vi "NiXnet GetSubProperty.vi"(6 "contextId":T1, 8 "error in":errorcluster, 9 "timeout (ms)":i32=-1, 10 "Request Data":T3, 11 "gRPC ID":T1) -> (0 "error out":errorcluster, 2 "Response Data":T2, 3 "gRPC ID out":T1)   [LabVIEW 2025, in "xnet-grpc_client.lvlib"]
uses:
  xnet-grpc_client.lvlib
  <vilib>/gRPC/LabVIEW gRPC Library/Shared/grpcId.ctl
  RPC Messages/nixnet_grpc_GetSubPropertyRequest.ctl
  RPC Messages/nixnet_grpc_GetSubPropertyRequest_subproperty_id_enum/nixnet_grpc_GetSubPropertyRequest_subproperty_id_enum.lvclass
  RPC Messages/nidevice_grpc_Session.ctl
  RPC Messages/nixnet_grpc_GetSubPropertyResponse.ctl
  RPC Messages/nixnet_grpc_GetSubPropertyResponse_property_value/nixnet_grpc_GetSubPropertyResponse_property_value.lvclass
  RPC Messages/nixnet_grpc_GetSubPropertyResponse_Flat.ctl
  RPC Messages/nixnet_grpc_GetSubPropertyRequest_subproperty_id_enum/nixnet_grpc_GetSubPropertyRequest_subproperty_id_enum.lvclass/nixnet_grpc_GetSubPropertyRequest_subproperty_id_enum.ctl
  RPC Messages/nixnet_grpc_GetSubPropertyResponse_property_value/nixnet_grpc_GetSubPropertyResponse_property_value.lvclass/nixnet_grpc_GetSubPropertyResponse_property_value.ctl
  14035477-4c25-4107-8ed5-d0c4ef420ce5.vi
  RPC Messages/RichToFlatnidevice_grpc_Session.vi
  RPC Messages/nixnet_grpc_GetSubPropertyRequest_subproperty_id_enum/GetActiveFieldIndex.vi
  RPC Messages/nixnet_grpc_GetSubPropertyRequest_subproperty_id_enum/Getproperty_id.vi
  RPC Messages/nixnet_grpc_GetSubPropertyRequest_subproperty_id_enum/Getproperty_id_raw.vi
  <vilib>/gRPC/LabVIEW gRPC Library/Shared/TranslateGrpcError.vi
  <vilib>/gRPC/LabVIEW gRPC Library/Shared/Wait On Occurrence Wrapper.vi
  RPC Messages/nixnet_grpc_GetSubPropertyResponse_property_value/Setu32_scalar.vi
  RPC Messages/nixnet_grpc_GetSubPropertyResponse_property_value/Setstr.vi
  RPC Messages/nixnet_grpc_GetSubPropertyResponse_property_value/Setf64_scalar.vi
  <vilib>/gRPC/LabVIEW gRPC Library/Shared/Wait On Occurence.vi
  <vilib>/gRPC/LabVIEW gRPC Library/Server API/Server/Get Server DLL Path.vi
  <vilib>/Utility/error.llb/Error Cluster From Error Code.vi
  <vilib>/Utility/config.llb/Open Config Data.vi
  <vilib>/Utility/config.llb/Write Key.vi
  <vilib>/Utility/config.llb/Write Key (Boolean).vi
  <vilib>/Utility/config.llb/Not A Config Data Refnum.vi
  <vilib>/Utility/config.llb/Read Key.vi
  <vilib>/Utility/config.llb/Read Key (Boolean).vi
  <vilib>/Utility/config.llb/Close Config Data.vi
  RPC Messages/nixnet_grpc_GetSubPropertyResponse_property_value/GetActiveFieldName.vi
  <vilib>/gRPC/LabVIEW gRPC Library/grpc-lvsupport-release.lvlib
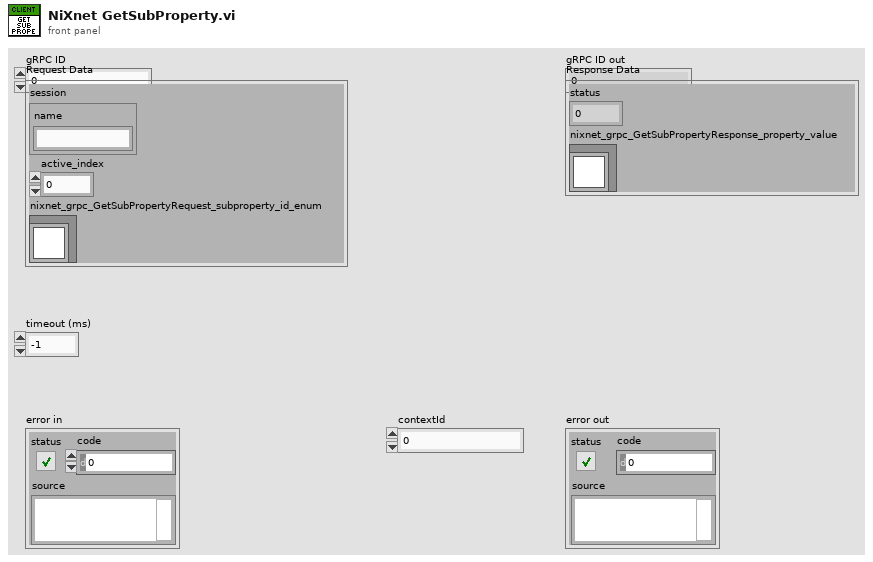
[diagram p1: front panel]
types:
  T1 = typedef "grpc-lvsupport-release.lvlib/grpcId.ctl" = u64
  T2 = typedef "xnet-grpc_client.lvlib/nixnet_grpc_GetSubPropertyResponse.ctl" = cluster{"status":i32, "nixnet_grpc_GetSubPropertyResponse_property_value":refnum<class "nixnet_grpc_GetSubPropertyResponse_property_value.lvclass">}
  T3 = typedef "xnet-grpc_client.lvlib/nixnet_grpc_GetSubPropertyRequest.ctl" = cluster{"session":T4, "active_index":u32, "nixnet_grpc_GetSubPropertyRequest_subproperty_id_enum":refnum<class "nixnet_grpc_GetSubPropertyRequest_subproperty_id_enum.lvclass">}
  T4 = typedef "xnet-grpc_client.lvlib/nidevice_grpc_Session.ctl" = cluster{"name":string}
  T5 = typedef "xnet-grpc_client.lvlib/nixnet_grpc_GetSubPropertyResponse_Flat.ctl" = cluster{"status":i32, "nixnet_grpc_GetSubPropertyResponse_property_value_selected_index":i32, "u32_scalar":u32, "str":string, "f64_scalar":dbl}
  T6 = typedef "xnet-grpc_client.lvlib/nixnet_grpc_GetSubPropertyRequest_Flat.ctl" = cluster{"session":T7, "active_index":u32, "nixnet_grpc_GetSubPropertyRequest_subproperty_id_enum_selected_index":i32, "property_id":T8, "property_id_raw":u32}
  T7 = typedef "xnet-grpc_client.lvlib/nidevice_grpc_Session_Flat.ctl" = cluster{"name":string}
  T8 = typedef "xnet-grpc_client.lvlib/nixnet_grpc_SubProperty.ctl" = enum32{"SUB_PROPERTY_UNSPECIFIED", "SUB_PROPERTY_SESSION_SUB_CAN_START_TIME_OFF", "SUB_PROPERTY_SESSION_SUB_CAN_TX_TIME", "SUB_PROPERTY_SESSION_SUB_LIN_TX_N_CORRUPTED_CHKSUMS", "SUB_PROPERTY_SESSION_SUB_OUTPUT_QUEUE_UPDATE_FREQ", "SUB_PROPERTY_SESSION_SUB_J1939_ADDR_FILTER", "SUB_PROPERTY_SESSION_SUB_SKIP_N_CYCLIC_FRAMES"}
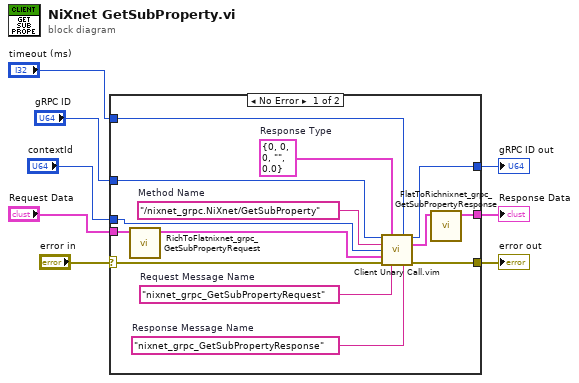
[diagram p0: block diagram]
diagram:
  n1 = case shown="No Error" "error in" {
    selector: "error in" -> [w18 w23]
    tunnel: [w17 w23] -> w7
    tunnel: "gRPC ID" -> [w16 w24]
    tunnel: [w15 w24] -> w5
    tunnel: "Request Data" -> [w12 _]
    tunnel: [w9 _] -> w3
    tunnel: "timeout (ms)" -> [w14 _]
    tunnel: "contextId" -> [w13 _]
    frame No Error {
      w19 = "nixnet_grpc_GetSubPropertyResponse"  # Response Message Name
      w20 = "nixnet_grpc_GetSubPropertyRequest"  # Request Message Name
      w21 = T5 {"status"=0, "nixnet_grpc_GetSubPropertyResponse_property_value_selected_index"=0, "u32_scalar"=0, "str"="", "f64_scalar"=0.0}  # Response Type
      w22 = "/nixnet_grpc.NiXnet/GetSubProperty"  # Method Name
      n2 = call "RichToFlatnixnet_grpc_GetSubPropertyRequest.vi"("InputCluster"=w12) -> ("OutputCluster"=w11:T6)  [unwired: 10 in]
      n3 = call "Client Unary Call.vim"("ClientID in"=w16, "Response Type"=w21, "timeout (ms)"=w14, "Method Name"=w22, "contextId"=w13, "Request Data"=w11, "error in"=w18, "Request Message Name"=w20, "Response Message Name"=w19) -> ("ClientID out"=w15:u64, "Response Data"=w10:T5, "error out"=w17:errorcluster)  [unwired: 4 in]
      n4 = call "FlatToRichnixnet_grpc_GetSubPropertyResponse.vi"("InputCluster"=w10) -> ("OutputCluster"=w9:T2)  [unwired: 10 in]
    }
    frame Error {
    }
  }
  "error out" <- w7
  "gRPC ID out" <- w5
  "Response Data" <- w3
